vi "setROI.vi"(0 "FakeCamera in":refnum<class "ThorLabsCsCamera.lvclass">, 7 "Seperator":string, 9 "value":string, 11 "error in (no error)":errorcluster) -> (4 "FakeCamera out":refnum<class "ThorLabsCsCamera.lvclass">, 6 "output cluster":T1, 8 "value":dbl, 10 "Command out":string, 15 "error out":errorcluster)   [LabVIEW 2020, in "ThorLabsCsCamera.lvclass"]
uses:
  ThorLabsCsCamera/ThorLabsCsCamera.lvclass
  subVis/ROI_TypDef.ctl
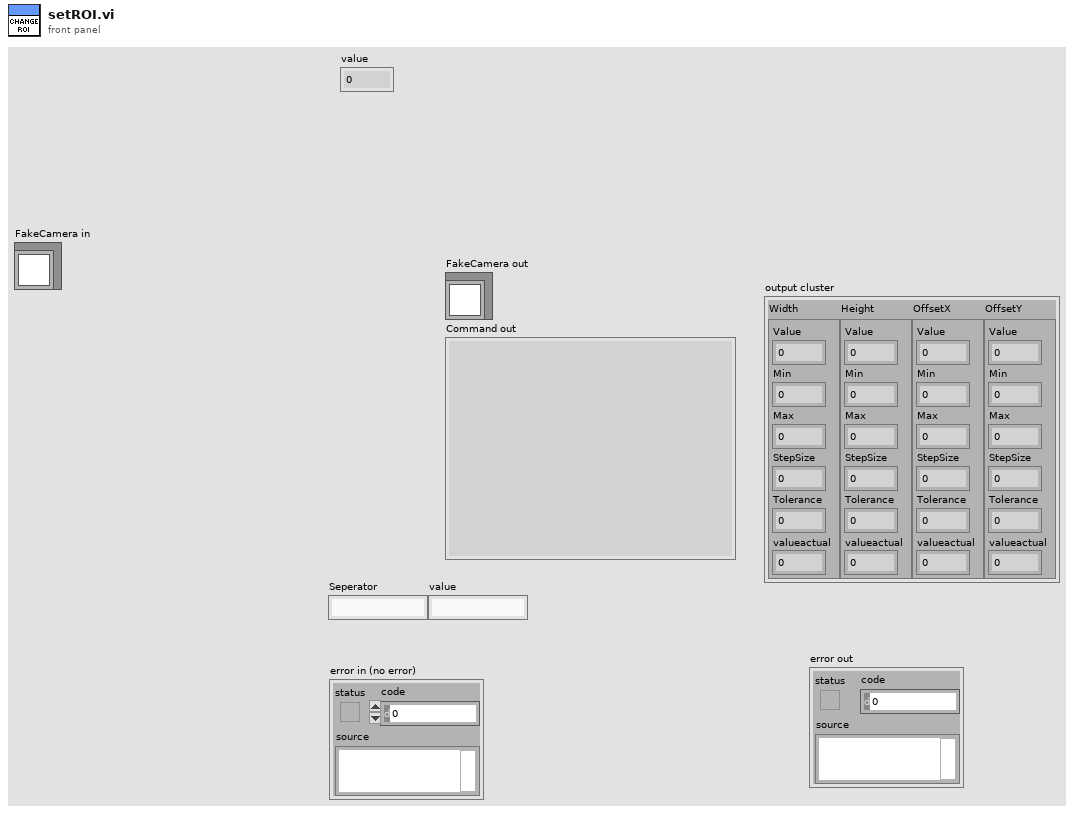
[diagram p1: front panel]
types:
  T1 = typedef "ROI_TypDef.ctl" = cluster{"Width":cluster{"Value":dbl, "Min":dbl, "Max":dbl, "StepSize":dbl, "Tolerance":dbl, "valueactual":dbl}, "Height":cluster{"Value":dbl, "Min":dbl, "Max":dbl, "StepSize":dbl, "Tolerance":dbl, "valueactual":dbl}, "OffsetX":cluster{"Value":dbl, "Min":dbl, "Max":dbl, "StepSize":dbl, "Tolerance":dbl, "valueactual":dbl}, "OffsetY":cluster{"Value":dbl, "Min":dbl, "Max":dbl, "StepSize":dbl, "Tolerance":dbl, "valueactual":dbl}}
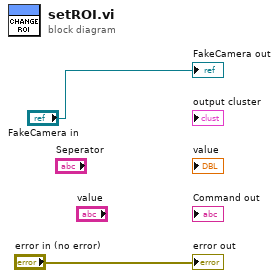
[diagram p0: block diagram]
diagram:
  "error out" <- "error in (no error)"
  "FakeCamera out" <- "FakeCamera in"
